vi "NXTServo-Remote.vi"() -> ()   [LabVIEW 2009]
uses:
  <vilib>/NXT/Block Support/NXT_InputPort.ctl
  <vilib>/NXT/Subs/LVHSConnector.ctl
panel:
  out "Voltage":u8
  in  "Speed":u8
  in  "Position":u16
  in  "Servo Number":u8
  in  "NXT":T1
  out "NXT dup":T1 caption="NXT"
  in  "Input Port":T2 items=["Port 1", "Port 2", "Port 3", "Port 4"]
  # "mindsensors.com\nCopyright (c) 2009 by mindsensors.com\nEmail: info (<at>) mindsensors (<dot>) com\n\nThis program is free software. You can redistribute it and/or modify\nit under the terms of the GNU General Public License as published by\nthe Free Software Foundation; version 3 of the License.\nRead the license at: http://www.gnu.org/licenses/gpl.txt"
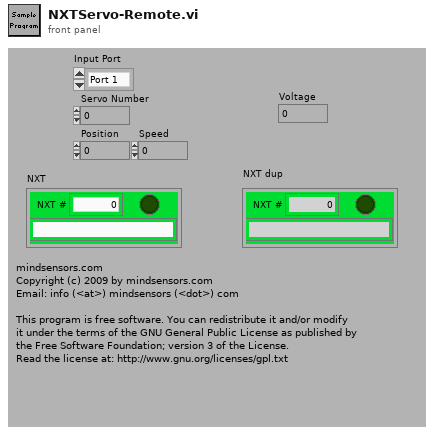
[diagram p1: front panel]
types:
  T1 = typedef "LVHSConnector.ctl" = cluster{"error":errorcluster, "address":string, "NXT #":i32, "Show Error":bool}
  T2 = typedef "NXT_InputPort.ctl" = u8
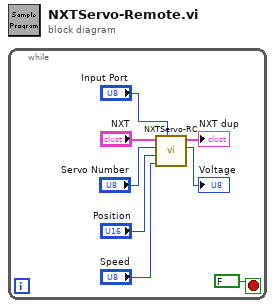
[diagram p0: block diagram]
diagram:
  n1 = while {
    stop <- FALSE stop-if-true
    n2 = call "NXTServo-RC.vi"("Input Port"="Input Port", "Speed"="Speed", "Position"="Position", "Servo Number"="Servo Number", "NXT"="NXT") -> ("Voltage"=→"Voltage":u8, "NXT dup"=→"NXT dup":T1)  [unwired: 4 in, 1 out]
  }
